vi "nominal ingest job get.vi"(8 "error in (no error)":errorcluster, 9 "out_job":i32, 10 "rid":string, 11 "client":i32) -> (0 "error out":errorcluster, 1 "out_job out":i32, 3 "function return":i32)   [LabVIEW 2020, in "client.lvlib"]
doc: "int32_t nominal_ingest_job_get(int32_t client, const char *rid, int32_t *out_job);"
uses:
  client.lvlib
  bin/nominalClient_64.dll
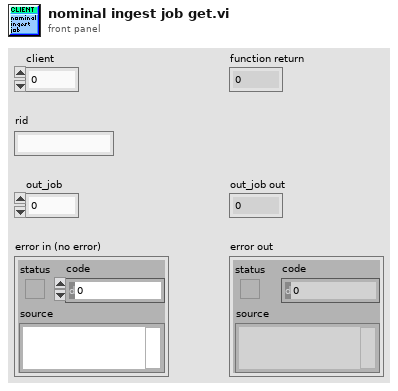
[diagram p1: front panel]
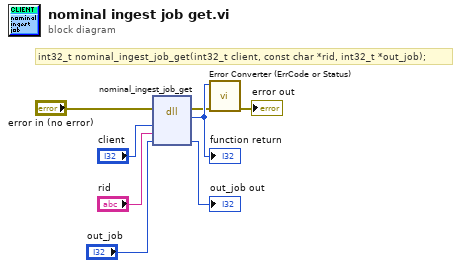
[diagram p0: block diagram]
diagram:
  # "int32_t nominal_ingest_job_get(int32_t client, const char *rid, int32_t *out_job);"
  n1 = dll-call lib="C:/code/labview-client-rs/lv_src/bin/nominalClient_*.*" fn="nominal_ingest_job_get"(error in="error in (no error)", "client"="client", "rid"="rid", "out_job"="out_job") -> (error out=w2:errorcluster, w8:i32, "out_job"=→"out_job out":i32)  [unwired: 4 in, 1 out]
  "function return" <- w8
  n2 = call "Error Converter (ErrCode or Status).vi"("error in (no error)"=w2, "error code"=w8) -> ("error out"=→"error out":errorcluster)  [unwired: 9 in]
